vi "RegisterNodeInfoEvent.vi"(8 "error in (no error)":errorcluster, 11 "handle":u64) -> (0 "error out":errorcluster, 3 "Node Info Event":refnum<user-event>)   [LabVIEW 2015, in "ReDeX.lvlib"]
doc: "redex_lv_result redex_lv_register_testpoint_info_event(redex_lv_handle handle,\n redex_lv_event_ref *ref);"
uses:
  ReDeX.lvlib
  C:/ReDeX/ReDeX.dll
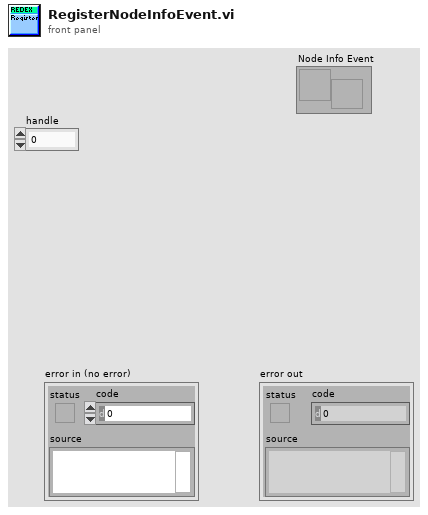
[diagram p1: front panel]
types:
  T1 = cluster{"Nodes":cluster{"ID":string, "Type":string}[]}
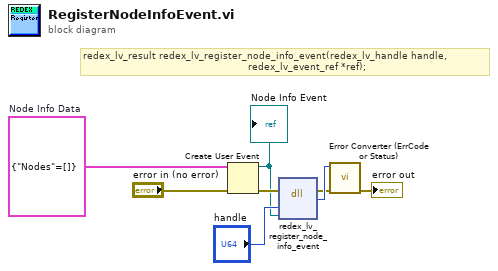
[diagram p0: block diagram]
diagram:
  w2 = T1 {"Nodes"=[]}  # Node Info Data
  # "redex_lv_result redex_lv_register_node_info_event(redex_lv_handle handle,\n                                                       redex_lv_event_ref *ref);"
  n1 = Create User Event(user event datatype=w2, error in="error in (no error)") -> (user event=w1:refnum<user-event>, error out=w3:errorcluster)
  "Node Info Event" <- w1
  n2 = dll-call lib="C:/ReDeX/ReDeX.dll" fn="redex_lv_register_node_info_event"(error in=w3, "handle"="handle", "ref"=w1) -> (error out=w7:errorcluster, "return type"=w8:u32)  [unwired: 4 in, 1 out]
  n3 = call "Error Converter (ErrCode or Status).vi"("error in (no error)"=w7, "error code"=w8) -> ("error out"=→"error out":errorcluster)  [unwired: 9 in]
